vi "GEOM_Check_optimize_time.vi"() -> (2 "optimize":bool)   [LabVIEW 2016]
uses:
  DBSHAND/private/vis/DatabaseHand_Element_Get(bool).vi
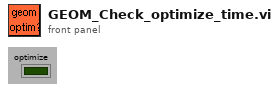
[diagram p1: front panel]
types:
  T1 = typedef "DatabaseHand_RefNum.ctl" = refnum<vi>
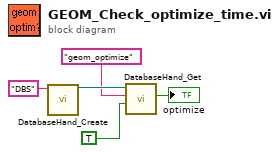
[diagram p0: block diagram]
diagram:
  n1 = call "DatabaseHand_Create.vi"("Name"="DBS") -> ("Database RefNum out"=w4:T1)  [unwired: 1 in, 9 out]
  n2 = call-poly "DatabaseHand_Get.vi"("default value"=TRUE, "name"="geom_optimize", "Database RefNum in"=w4) -> ("value"=→"optimize":bool)  [unwired: 2 in, 6 out]
